vi "ReadAttributes.vi"(8 "ErrorIn":errorcluster, 11 "YActorIn":refnum<class "YActor.lvclass">) -> (0 "ErrorOut":errorcluster, 3 "YActorOut":refnum<class "YActor.lvclass">)   [LabVIEW 2021, in "YActor.lvclass"]
uses:
  YActor.lvclass
  YActor.lvclass/YActor.ctl
  private/SendCommand.vi
  private/WaitForReply.vi
  private/CreateLocalVI.vi
  private/ExeuteInlineVI.vi
  private/GetRemoteVIRef.vi
  private/GetNameOfVI.vi
  QuickCast.vi
  SyncData.vi
  private/VINameProperty.vi
  private/MessageCounter.vi
  InlineReferencePool.vi
  private/ExecuteVI.vi
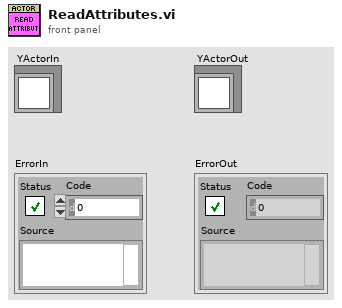
[diagram p1: front panel]
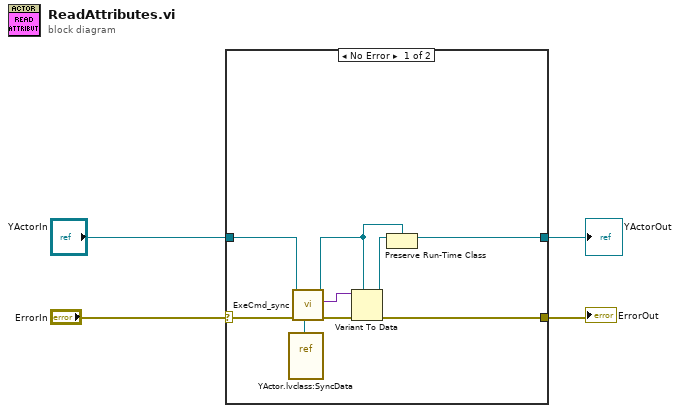
[diagram p0: block diagram]
diagram:
  n1 = case shown="No Error" "ErrorIn" {
    selector: "ErrorIn" -> [w13 w15]
    tunnel: [w11 w15] -> w3
    tunnel: "YActorIn" -> [w9 w14]
    tunnel: [w6 w14] -> w1
    frame No Error {
      n2 = vi-ref "YActor.lvclass:SyncData.vi"() -> (w10:refnum<vi>)
      n3 = call "ExeCmd_sync.vi"("CmdVIRef"=w10, "ErrorIn"=w13, "YActorIn"=w9) -> ("ErrorOut"=w12:errorcluster, "ReplyData"=w8:variant, "YActorOut"=w5:refnum<class "YActor.lvclass">)  [unwired: 6 in]
      n4 = Variant To Data(error in=w12, type=w5, Variant=w8) -> (data=w7:refnum<class "YActor.lvclass">, error out=w11:errorcluster)
      n5 = Preserve Run-Time Class(object in=w7, 2:w5) -> (object out=w6:refnum<class "YActor.lvclass">)  [unwired: 1 in, 1 out]
    }
    frame Error {
    }
  }
  "ErrorOut" <- w3
  "YActorOut" <- w1
